vi "Periodic Tasks.vi"(8 "error in":errorcluster) -> ()   [LabVIEW 2020]
doc: "This VI runs in parallel to other tasks. It can contain as many user-defined periodic loops as you need. These can carry out PID or other sorts of timed response."
uses:
  myStates.ctl
  <vilib>/Rock Robotics/WPI/DriverStation/WPI_DriverStationRobotMode2.ctl
  4913f956-5bda-4107-8571-b517f3ac16c4.vi
  <vilib>/Rock Robotics/WPI/Utilities/WPI_GetSetVariantRefNum.vi
  <vilib>/Rock Robotics/Network Tables/NT Read Variant.vi
  <vilib>/Rock Robotics/Network Tables/NT Write Number.vi
  <vilib>/Rock Robotics/Network Tables/NT Read Number.vi
  Robot Global Data.vi
  <vilib>/Rock Robotics/Network Tables/NT Write Numeric Array.vi
  <vilib>/Rock Robotics/Network Tables/NT Write Boolean Array.vi
  <vilib>/Comparison/Equal/Equal Functor/Equal Functor.lvclass
  <vilib>/Rock Robotics/Network Tables/NT Write String.vi
  <vilib>/Utility/Data Type/NI_Data Type.lvlib
panel:
  in  "Current State":string
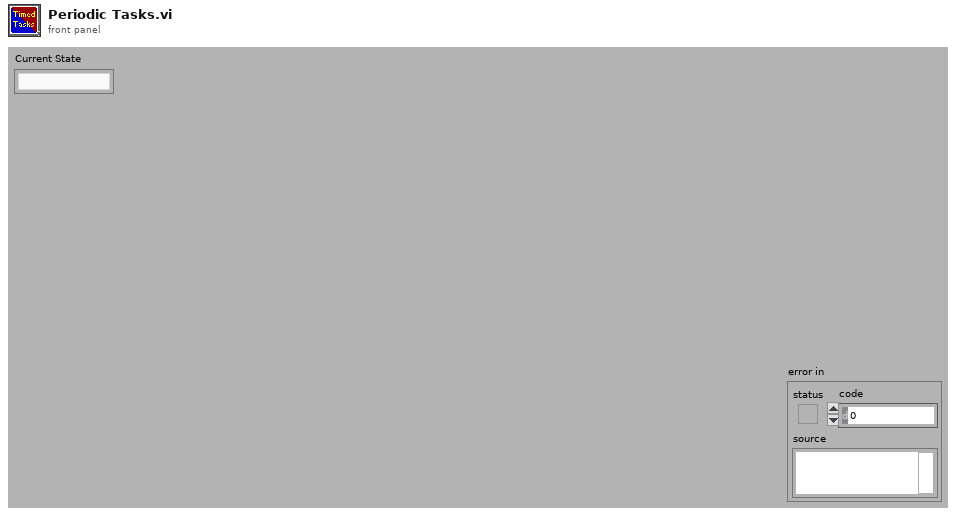
[diagram p1: front panel]
types:
  T1 = typedef "myStates.ctl" = enum16{"Init", "Manual Control", "Autonomous Traversal", "Avoid Left", "Avoid Right", "Return to Trench", "EXC Deploy", "EXC Excavate", "EXC Inch", "EXC Index", "EXC Retract", "Drive to Dep", "Approach Berm", "HAD Deploy", "HAD Deposit", "HAD Retract", "Return to EXC"}
  T2 = typedef "WPI_JoystickDevRef.ctl" = cluster{"Device":T3}
  T3 = typedef "WPI_JoystickDeviceEnum.ctl" = enum16{"USB 0", "USB 1", "USB 2", "USB 3", "USB 4", "USB 5"}
  T4 = typedef "WPI_RobotDriveDevRef.ctl" = cluster{"DevStatus":errorcluster, "Motors[]":T5[], "Square Inputs":bool, "Max Output":dbl}
  T5 = typedef "WPI_MotorControlDeviceRef.ctl" = cluster{"DeviceStatus":errorcluster, "Type":T6, "PWM":cluster{"PWM Channel":T7, "DeadBand":T8}, "CAN":cluster{"Device Number":u8, "SetOutput VI Ref":variant, "GetOutput VI Ref":variant, "Enable VI Ref":variant, "Disable VI Ref":variant, "Data":variant}, "Invert":bool, "DIO PWM":cluster{"PWM \"Enable\" Channel":T7, "DIOChannel":T9, "PWM Rate":dbl}}
  T6 = typedef "WPI_MotorControlType.ctl" = enum16{"PWM", "CAN", "DIO PWM"}
  T7 = typedef "FPGA_DIOPWMChannel.ctl" = enum8{"PWM 0", "PWM 1", "PWM 2", "PWM 3", "PWM 4", "PWM 5", "PWM 6", "PWM 7", "PWM 8", "PWM 9", "PWM MXP 0", "PWM MXP 1", "PWM MXP 2", "PWM MXP 3", "PWM MXP 4", "PWM MXP 5", "PWM MXP 6", "PWM MXP 7", "PWM MXP 8", "PWM MXP 9", "Invalid"}
  T8 = typedef "WPI_PWMDeadband.ctl" = cluster{"Name":string, "maxPositivePwm":i32, "minPositivePwm":i32, "centerPwm":i32, "maxNegativePwm":i32, "minNegativePwm":i32, "angularRange":u16}
  T9 = typedef "FPGA_DIOChannel.ctl" = enum8{"DIO 0", "DIO 1", "DIO 2", "DIO 3", "DIO 4", "DIO 5", "DIO 6", "DIO 7", "DIO 8", "DIO 9", "DIO MXP 0", "DIO MXP 1", "DIO MXP 2", "DIO MXP 3", "DIO MXP 4", "DIO MXP 5", "DIO MXP 6", "DIO MXP 7", "DIO MXP 8", "DIO MXP 9", "DIO MXP 10", "DIO MXP 11", "DIO MXP 12", "DIO MXP 13", "DIO MXP 14", "DIO MXP 15", "SPI Port CS1", "SPI Port CS2", "SPI Port CS3", "SPI Port MISO", "SPI Port MOSI", "Invalid"}
  T10 = cluster{"JoystickDevRef":T2, "RobotDriveDevRef":T4}
  T11 = typedef "WPI_DriverStationRobotMode2.ctl" = enum16{"Autonomous Disabled", "Autonomous Enabled", "Teleop Disabled", "Teleop Enabled", "Disconnected", "Finish", "Test Disabled", "Test Enabled", "Emergency Stopped"}
  T12 = cluster{"Axes[0]":dbl, "Axes[1]":dbl, "Axes[2]":dbl, "Axes[3]":dbl, "Axes[4]":dbl, "Axes[5]":dbl, "Axes[6]":dbl, "Axes[7]":dbl, "Axes[8]":dbl}
  T13 = cluster{"Buttons[0]":bool, "Buttons[1]":bool, "Buttons[2]":bool, "Buttons[3]":bool, "Buttons[4]":bool, "Buttons[5]":bool, "Buttons[6]":bool, "Buttons[7]":bool, "Buttons[8]":bool}
  T14 = typedef "WPI_AnalogChannelDevRef.ctl" = cluster{"DevStatus":errorcluster, "Analog Channel":T15}
  T15 = typedef "FPGA_AIChannel.ctl" = enum8{"AI 0", "AI 1", "AI 2", "AI 3", "AI MXP 0", "AI MXP 1", "AI MXP 2", "AI MXP 3", "Invalid"}
  T16 = typedef "WPI_DigitalOutputDevRef.ctl" = cluster{"DIO Channel":T9, "DevStatus":errorcluster}
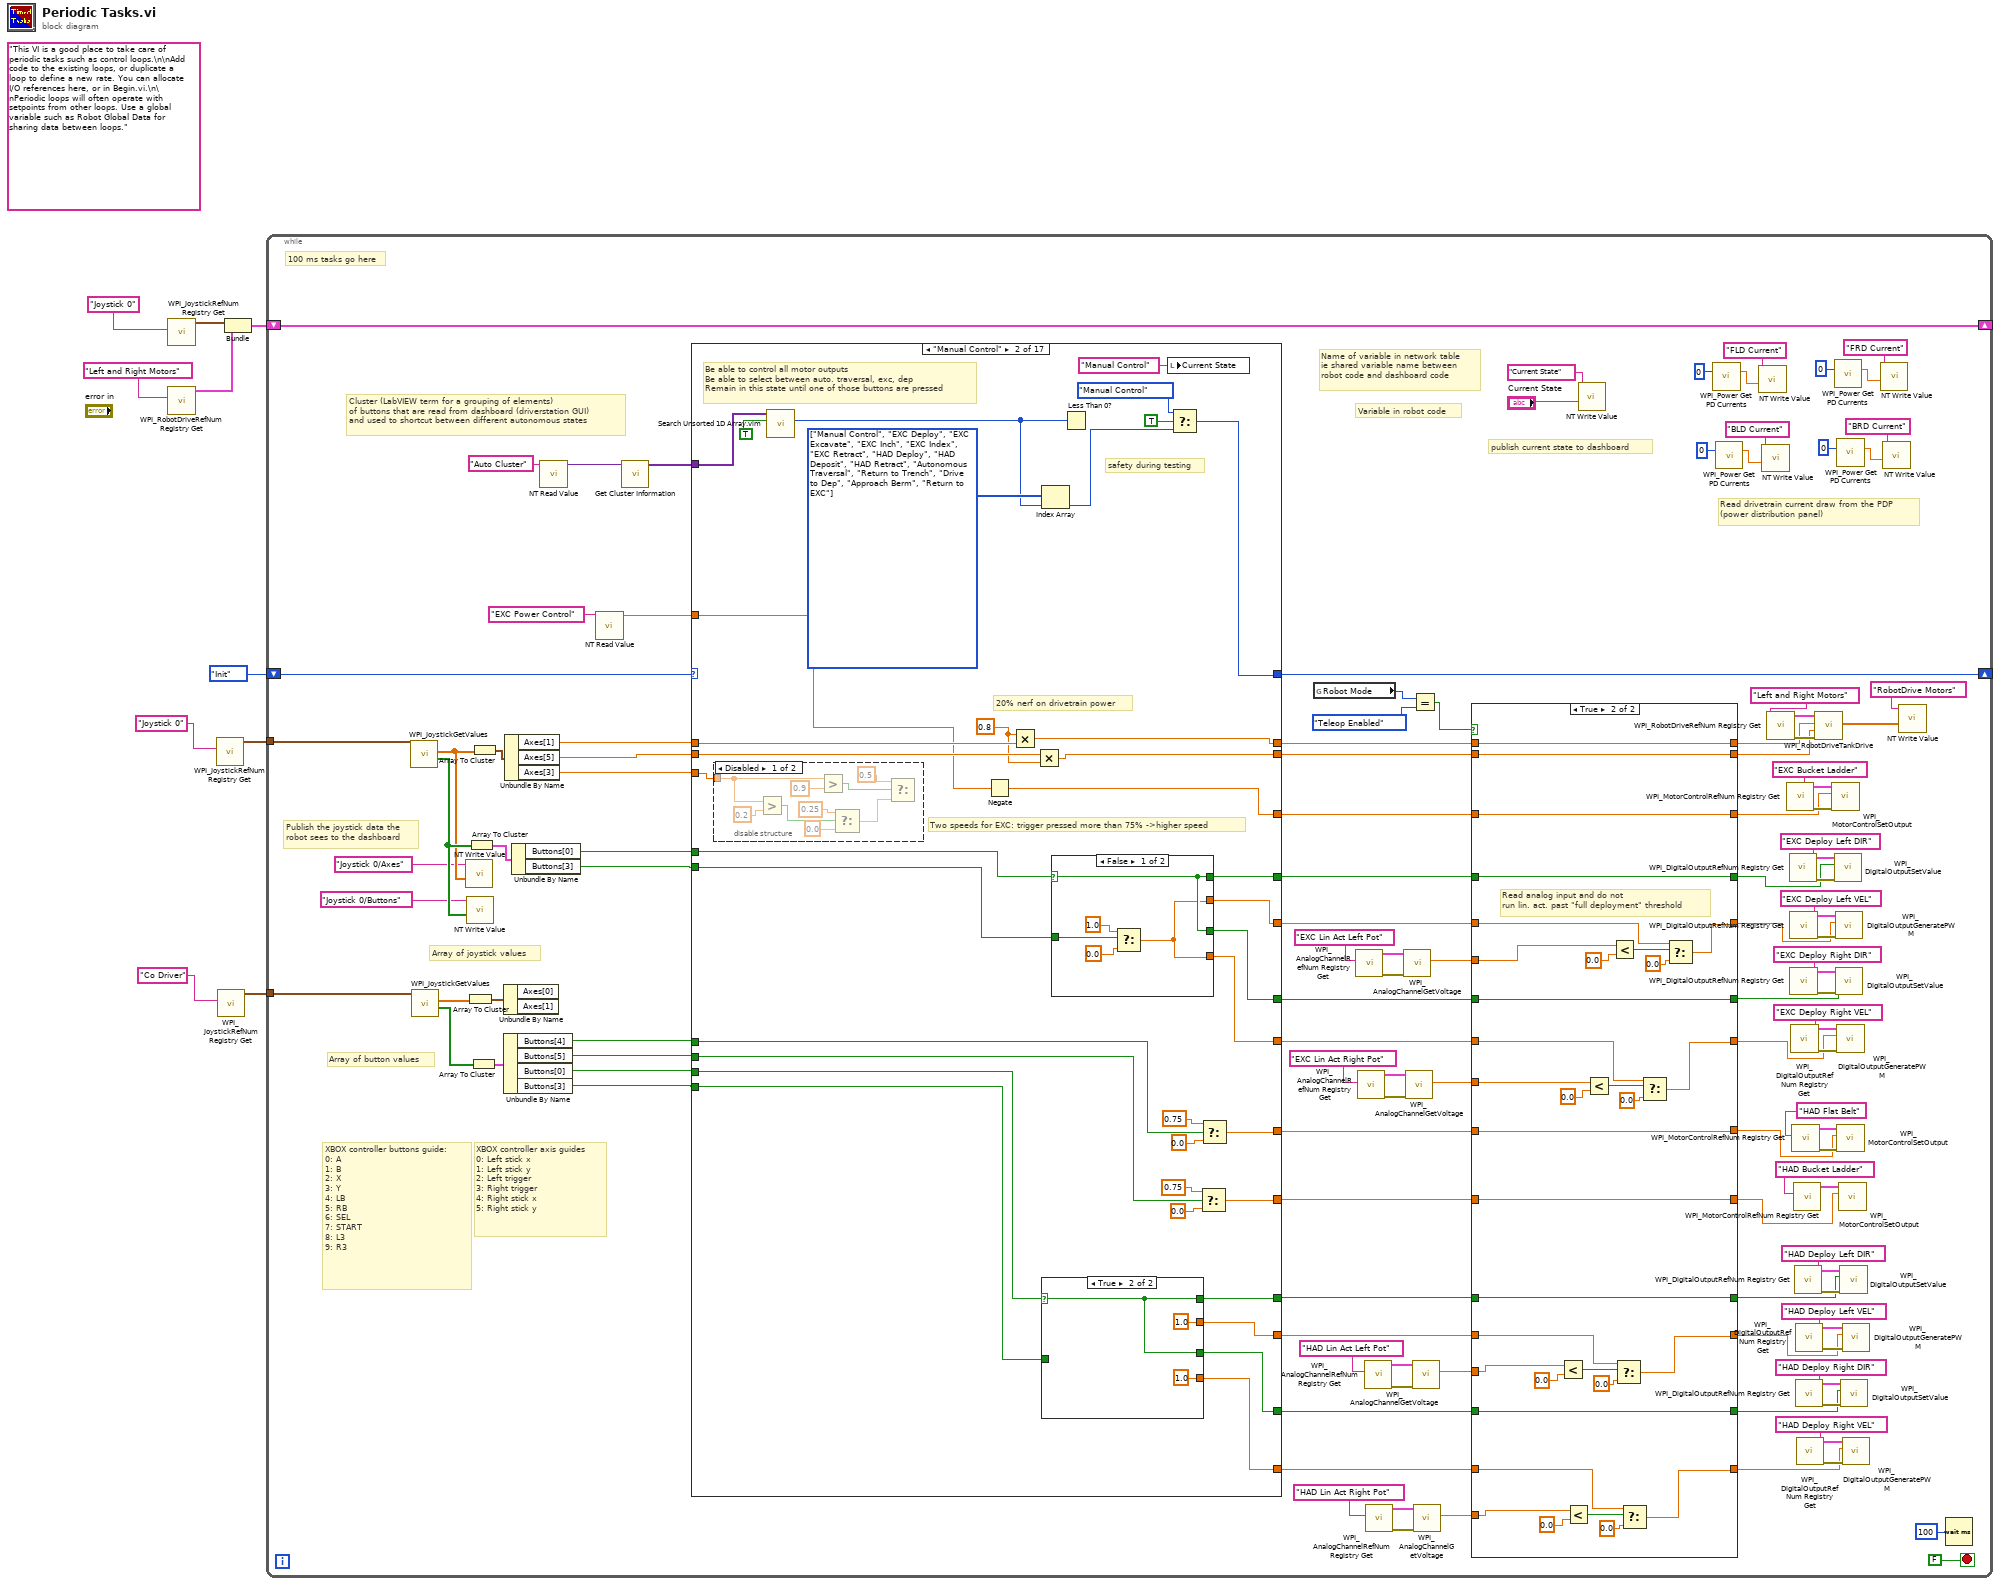
[diagram p0: block diagram]
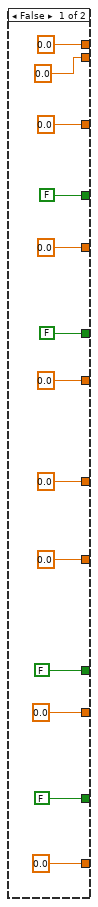
[diagram p2: hidden frame]
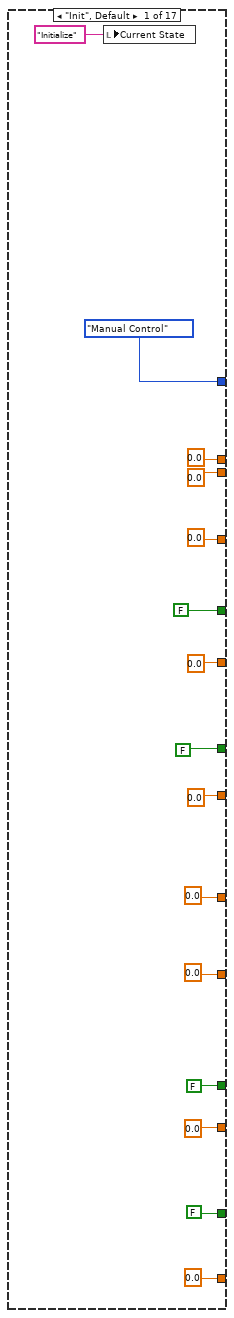
[diagram p3: hidden frame]
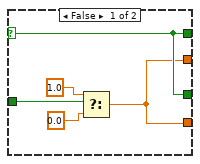
[diagram p5: hidden frame]
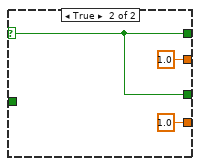
[diagram p6: hidden frame]
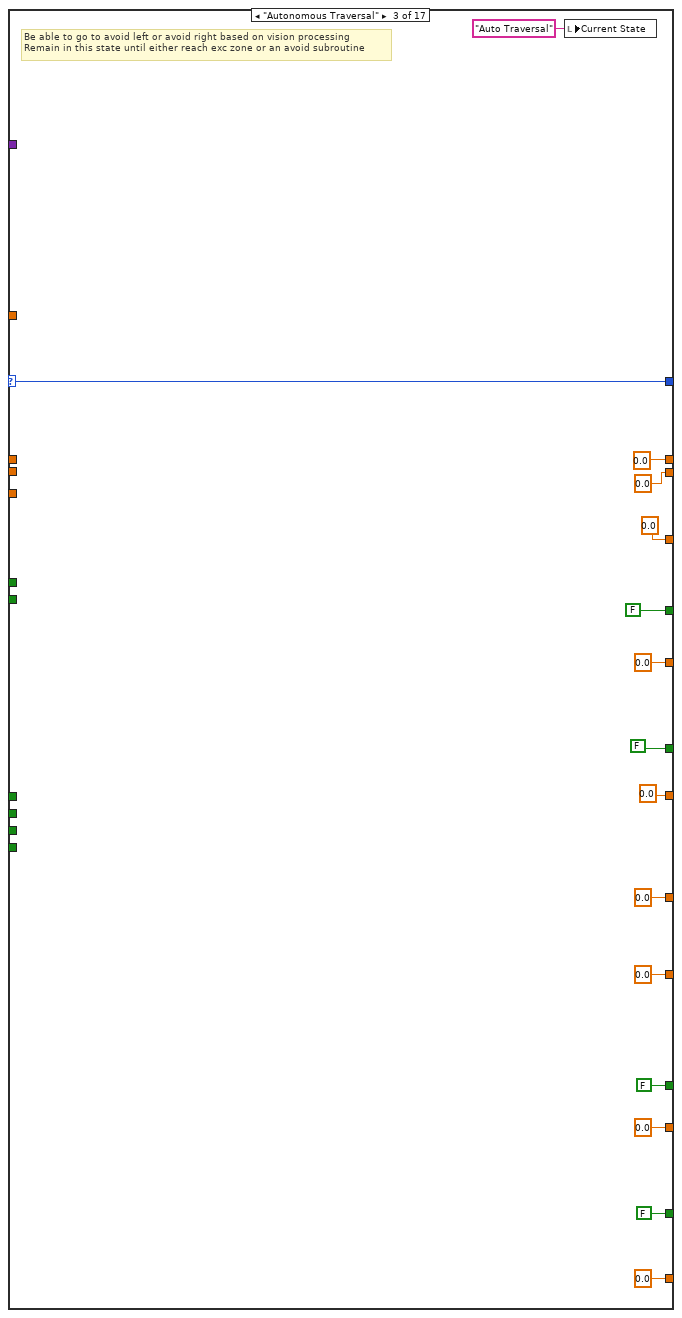
[diagram p7: hidden frame]
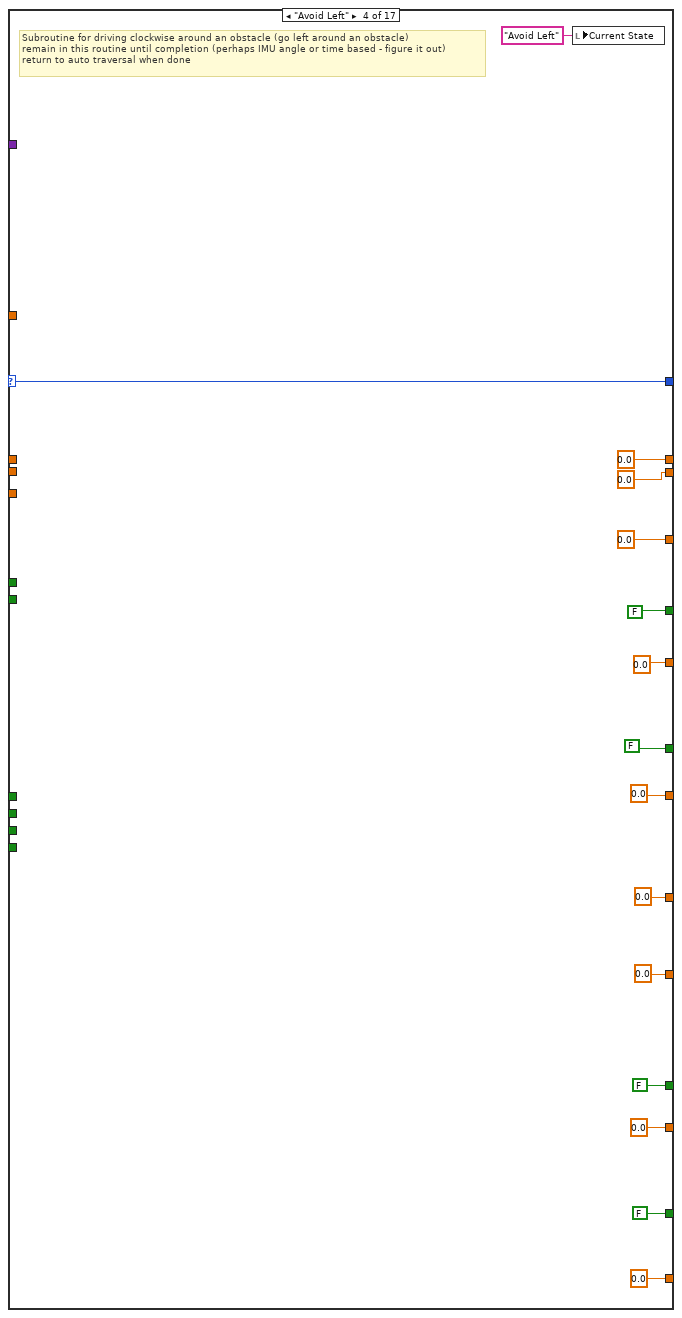
[diagram p8: hidden frame]
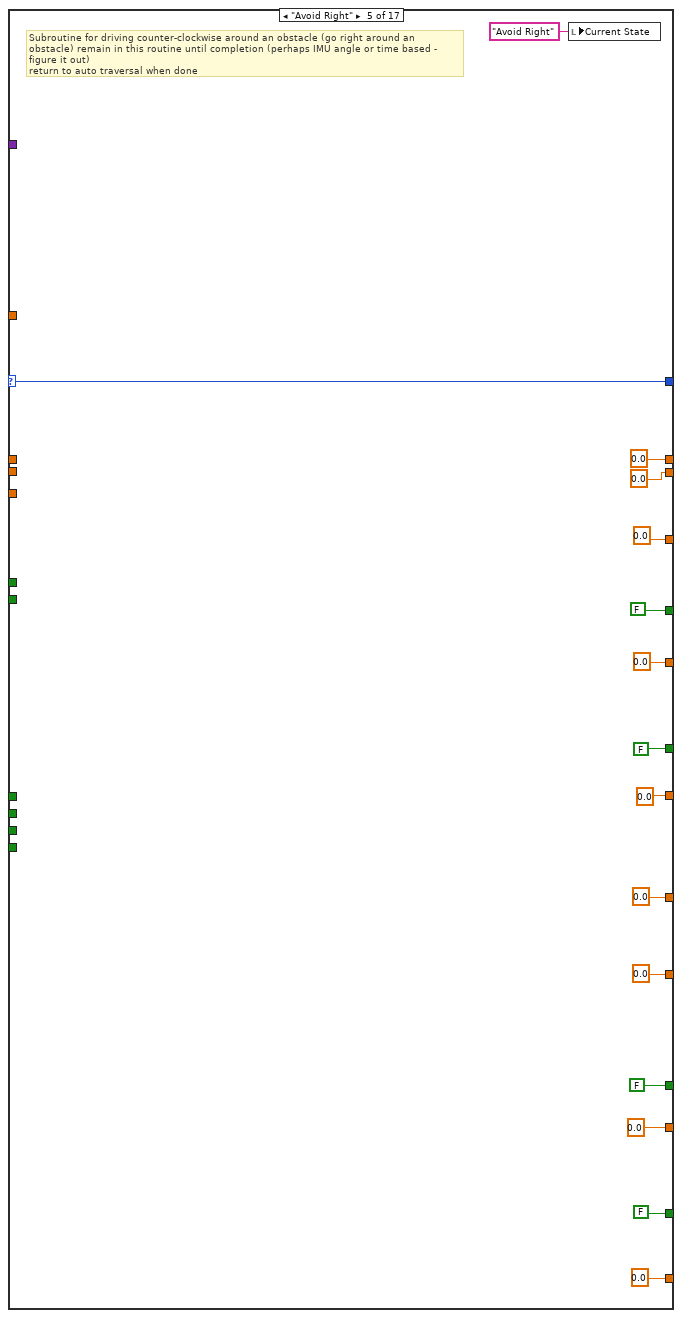
[diagram p9: hidden frame]
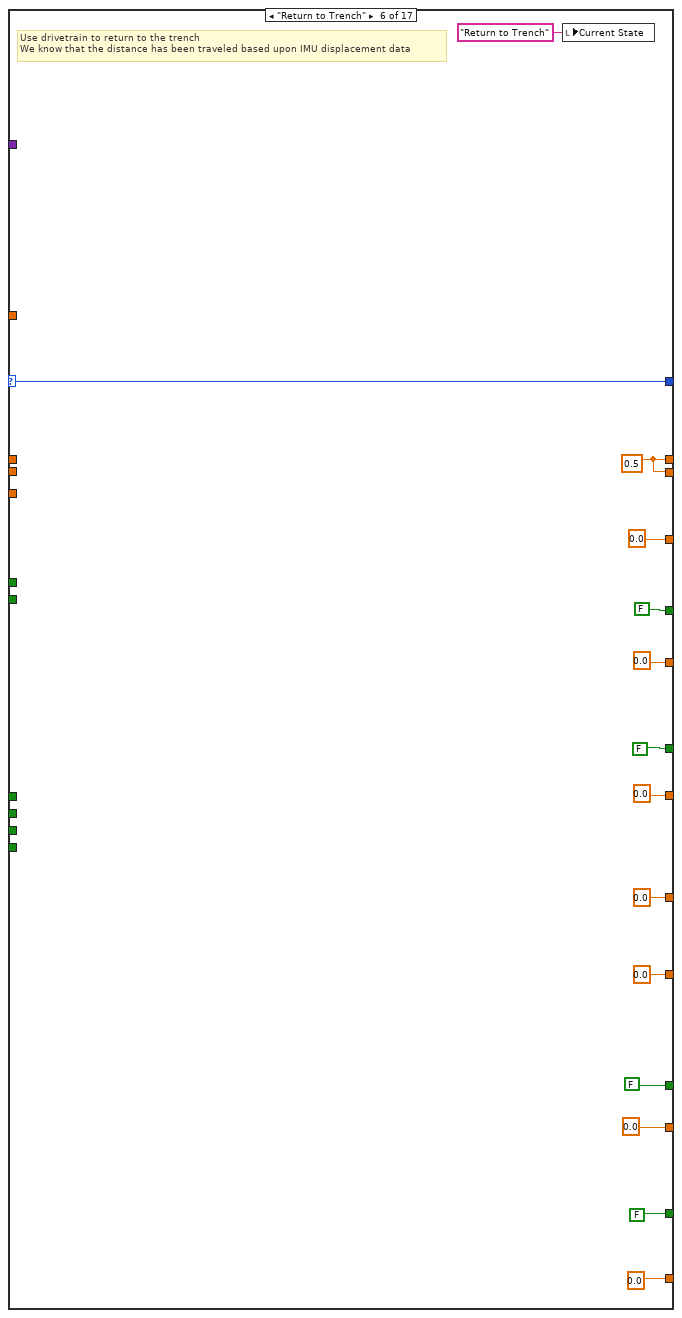
[diagram p10: hidden frame]
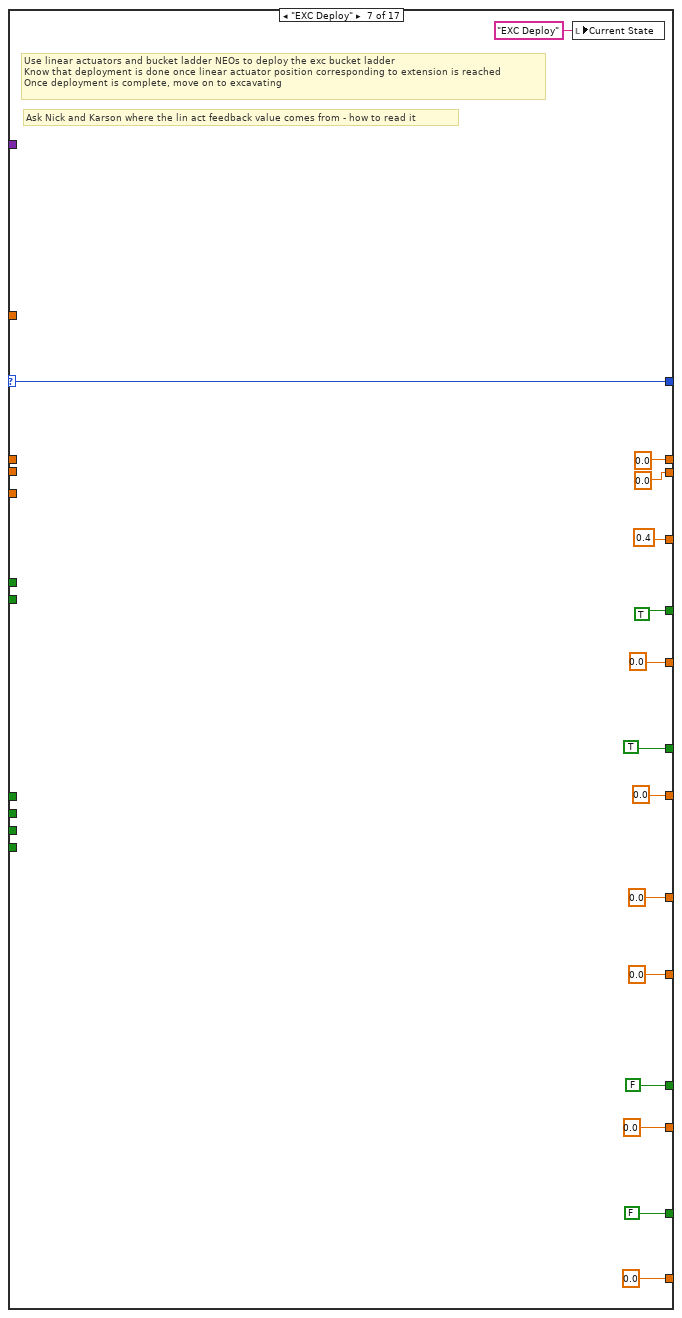
[diagram p11: hidden frame]
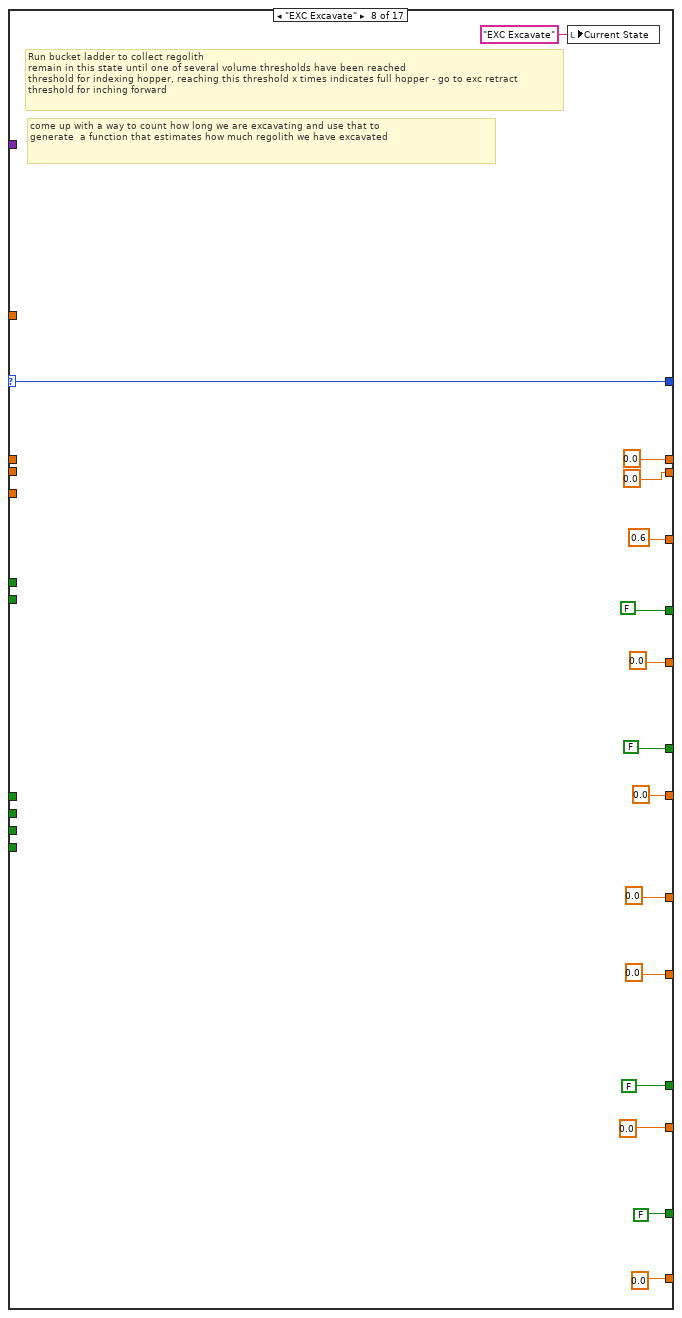
[diagram p12: hidden frame]
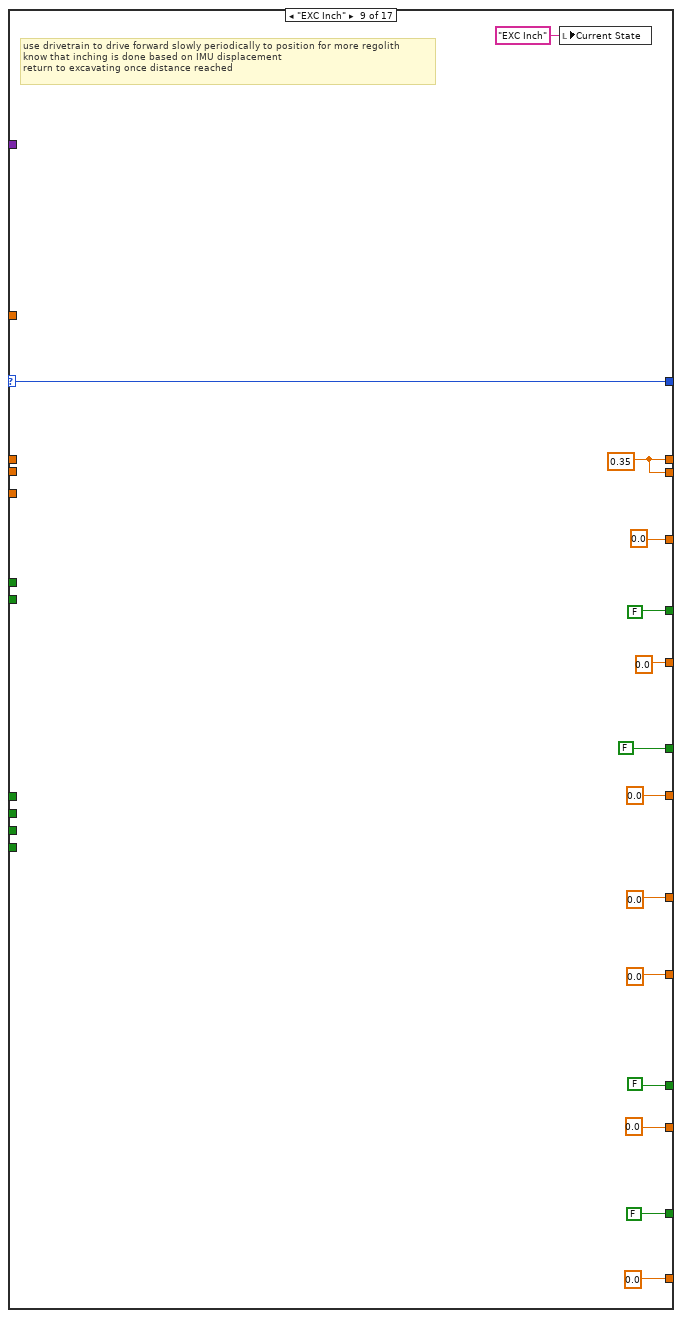
[diagram p13: hidden frame]
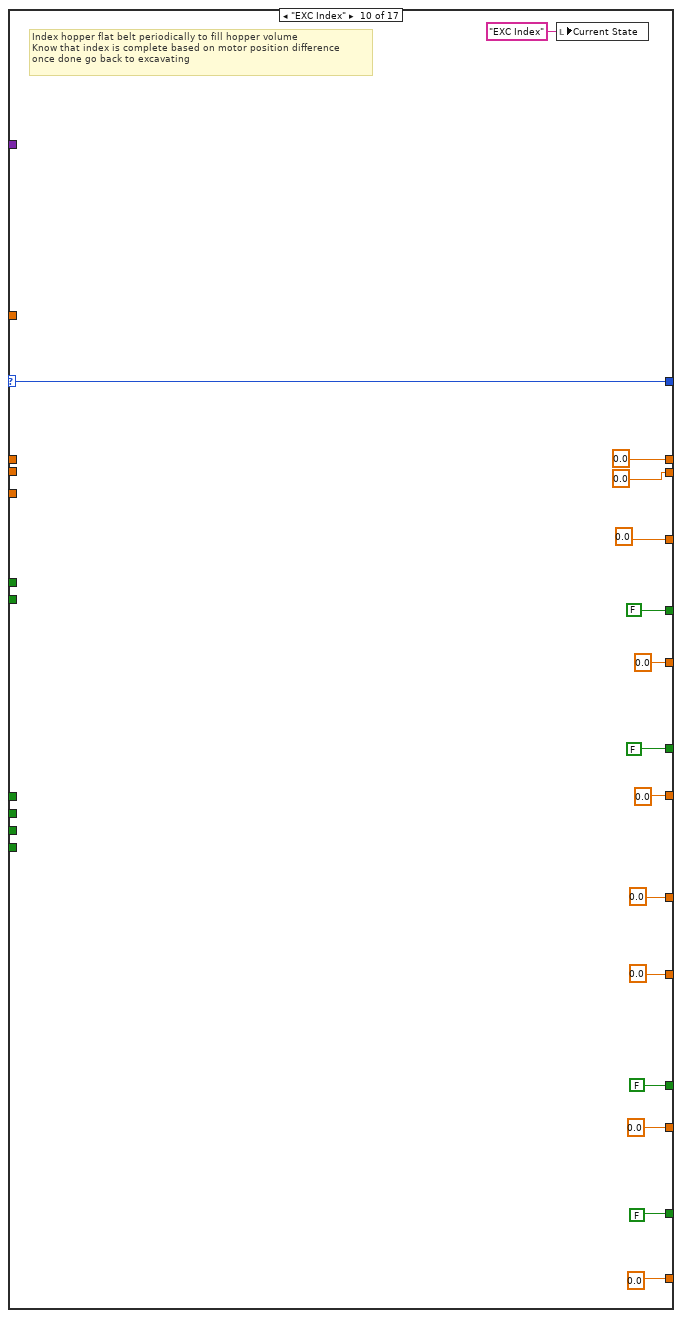
[diagram p14: hidden frame]
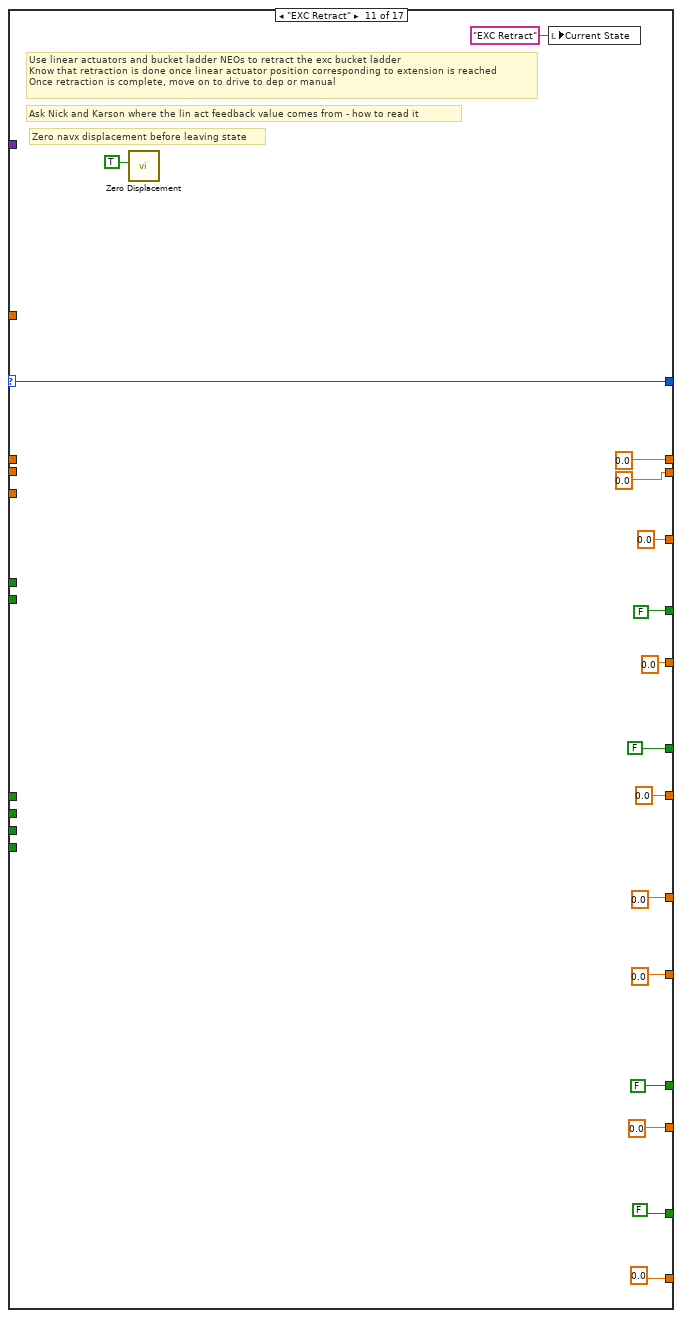
[diagram p15: hidden frame]
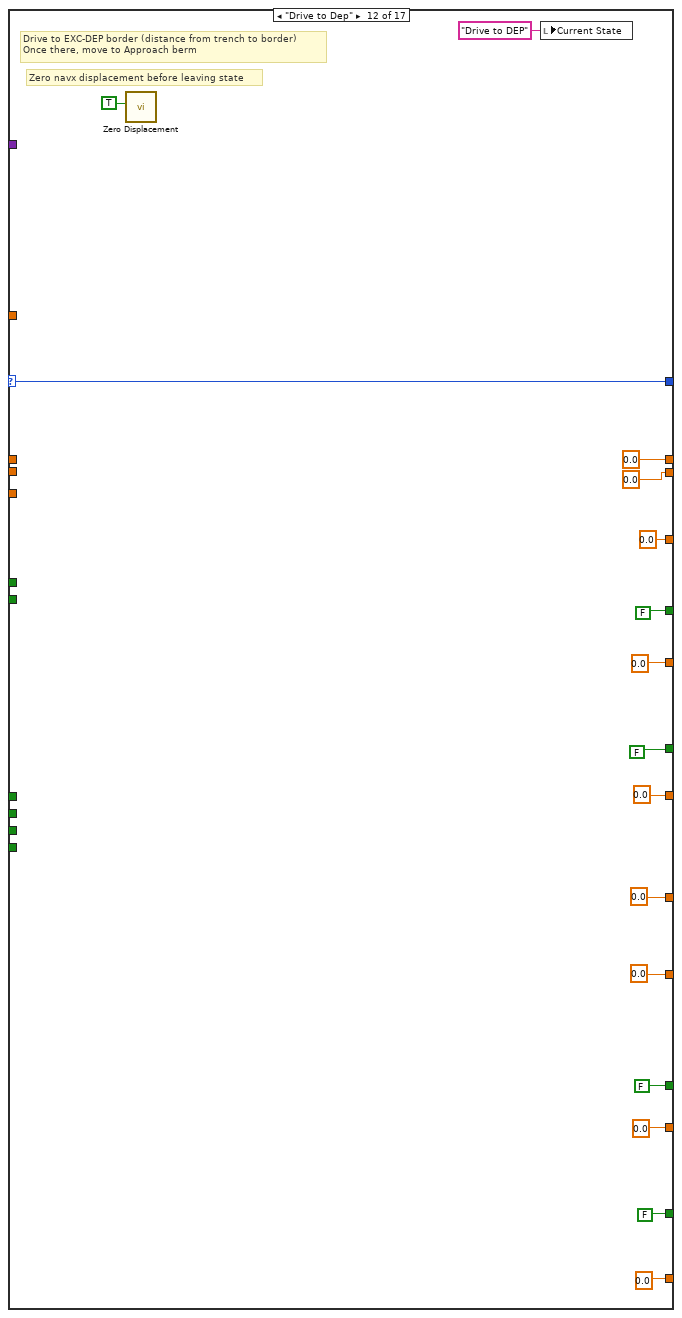
[diagram p16: hidden frame]
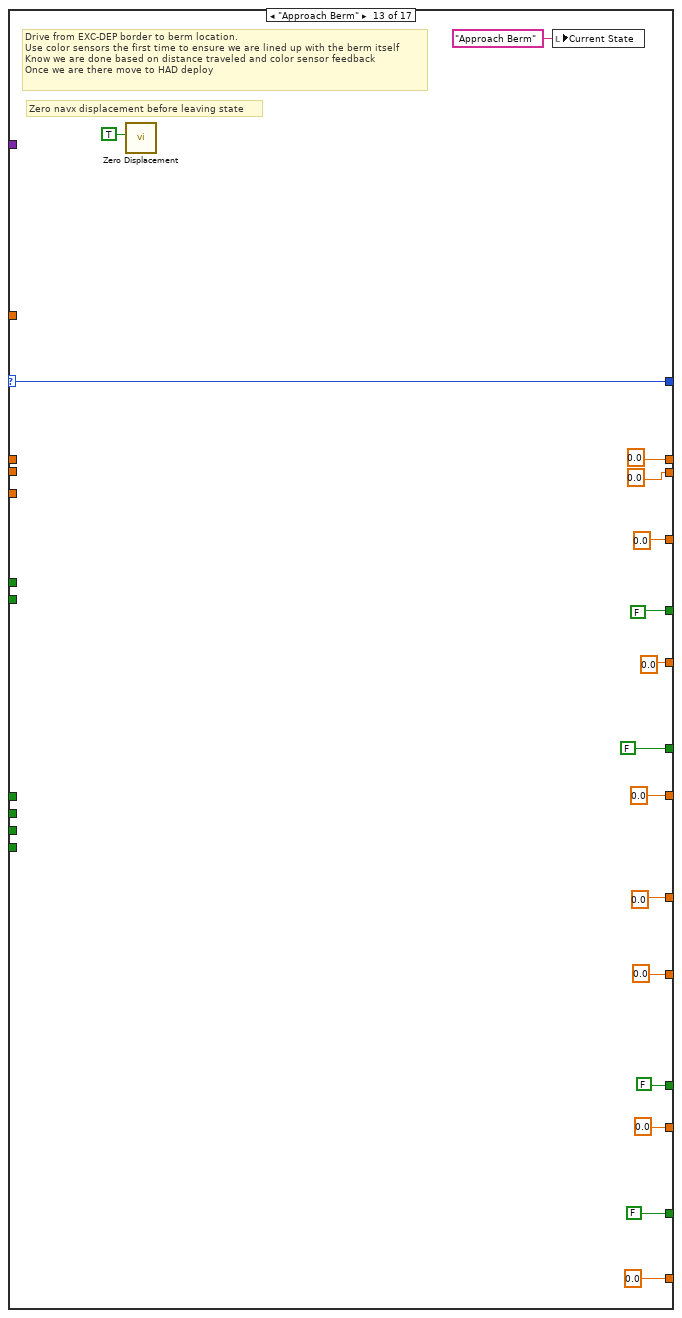
[diagram p17: hidden frame]
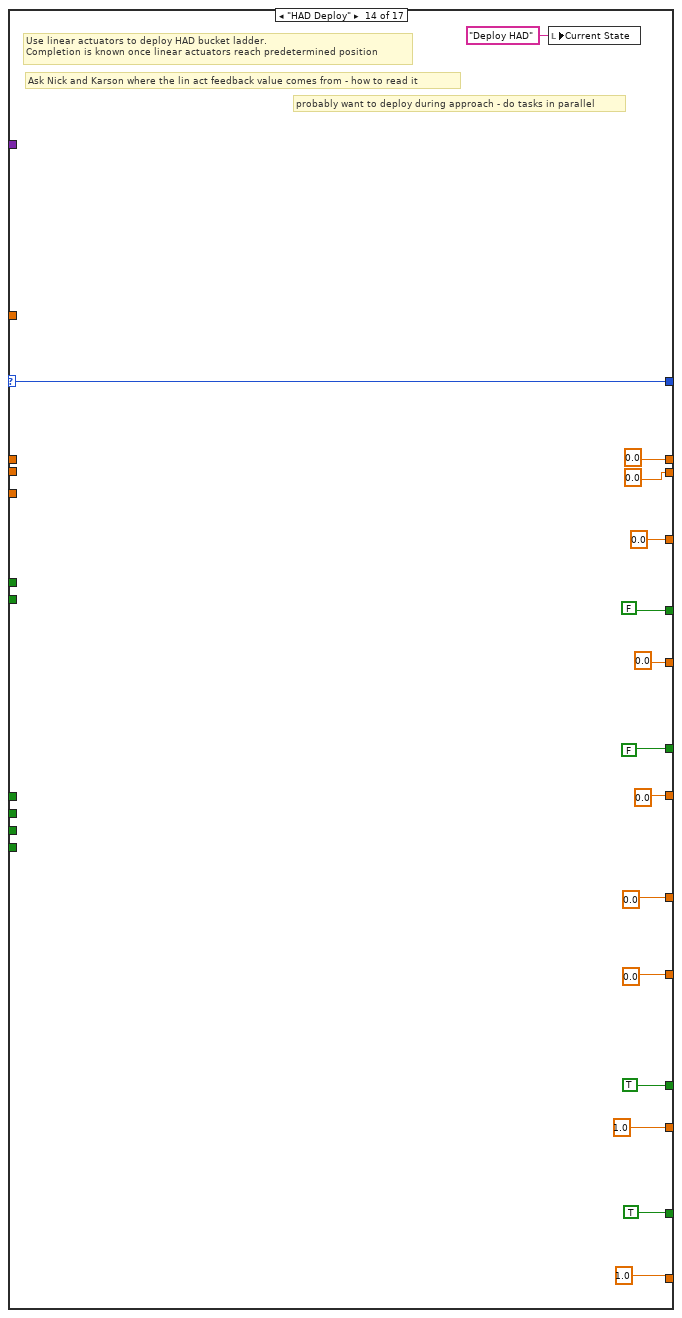
[diagram p18: hidden frame]
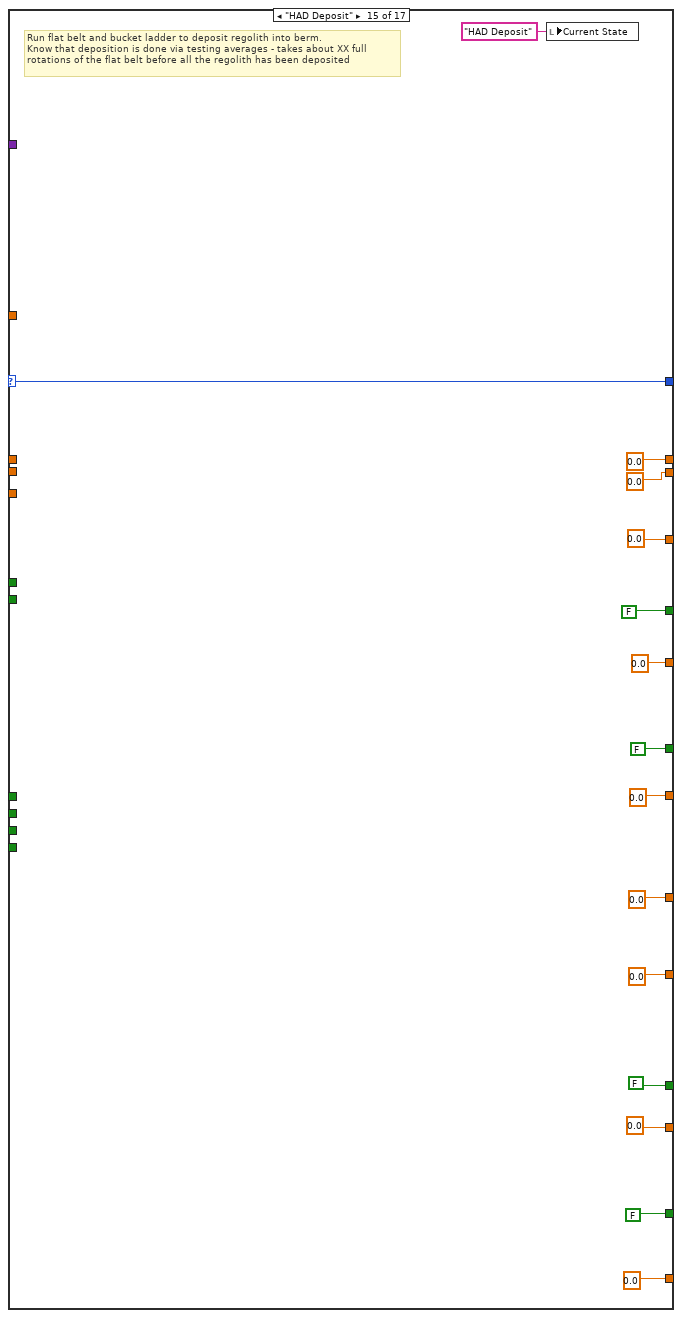
[diagram p19: hidden frame]
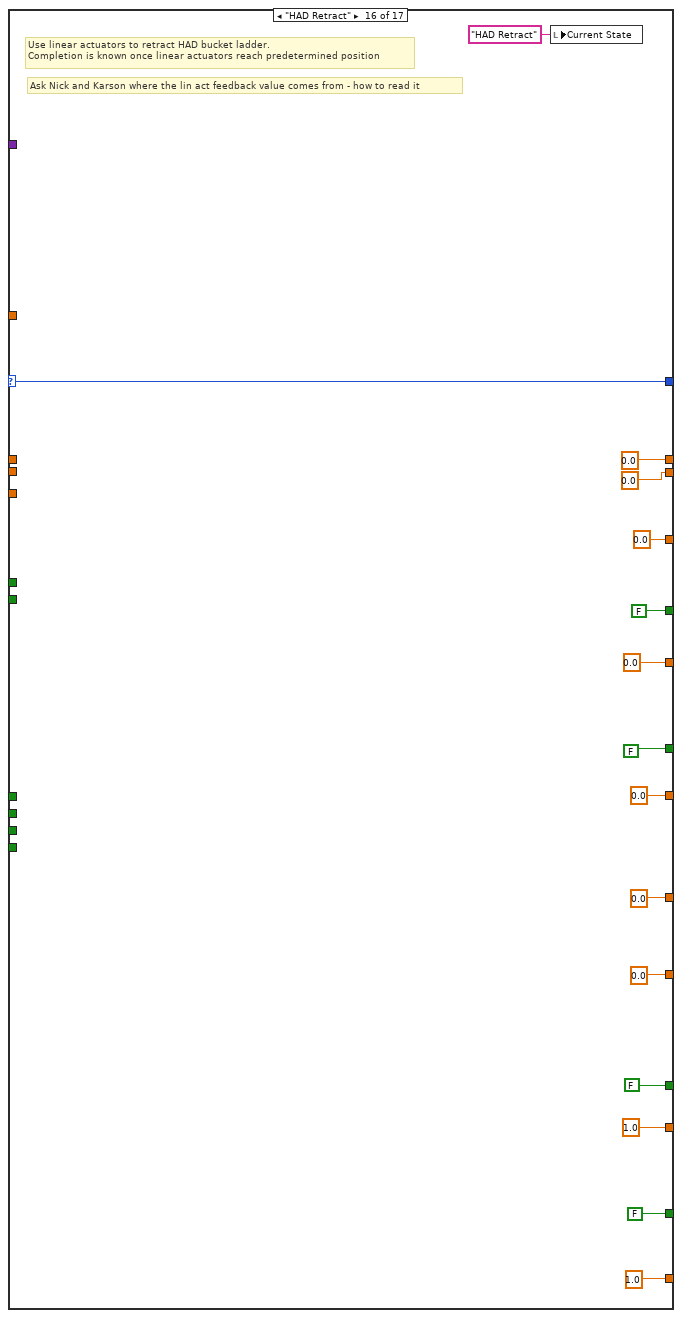
[diagram p20: hidden frame]
diagram:
  (unwired) "This VI is a good place to take care of periodic tasks such as control loops.\n\nAdd code to the existing loops, or duplicate a loop to define a new rate. You can allocate I/O references here, or in Begin.vi.\n\nPeriodic loops will often operate with setpoints from other loops. Use a global variable such as Robot Global Data for sharing data between loops."
  n1 = call <vilib>:"WPI_JoystickRefNum Registry Get.vi"("refnum name"="Joystick 0") -> ("JoystickDevRef"=w8:T2)  [unwired: 1 in, 9 out]
  n2 = call <vilib>:"WPI_RobotDriveRefNum Registry Get.vi"("refnum name"="Left and Right Motors") -> ("RobotDriveDevRef"=w7:T4)  [unwired: 1 in, 9 out]
  n3 = call <vilib>:"WPI_JoystickRefNum Registry Get.vi"("refnum name"="Joystick 0") -> ("JoystickDevRef"=w3:T2)  [unwired: 1 in, 9 out]
  n4 = call <vilib>:"WPI_JoystickRefNum Registry Get.vi"("refnum name"="Co Driver") -> ("JoystickDevRef"=w1:T2)  [unwired: 1 in, 9 out]
  n5 = Bundle("JoystickDevRef"=w8, "RobotDriveDevRef"=w7) -> (w6:T10)  [unwired: 1 out]
  n6 = while {
    shift-right: [w75] -> _
    shift-left: w6 -> [w75]
    shift-right: [w76] -> _
    shift-left: myStates."Init" -> [w77]
    tunnel: w3 -> [w74]
    tunnel: w1 -> [w73]
    stop <- FALSE stop-if-true
    # "Variable in robot code"
    # "Name of variable in network table\nie shared variable name between\nrobot code and dashboard code"
    # "publish current state to dashboard"
    # "Read drivetrain current draw from the PDP\n(power distribution panel)"
    # "XBOX controller axis guides\n0: Left stick x\n1: Left stick y\n2: Left trigger\n3: Right trigger\n4: Right stick x\n5: Right stick y"
    # "XBOX controller buttons guide:\n0: A\n1: B\n2: X\n3: Y\n4: LB\n5: RB\n6: SEL\n7: START\n8: L3\n9: R3"
    # "Array of joystick values"
    # "Array of button values"
    # "Cluster (LabVIEW term for a grouping of elements)\nof buttons that are read from dashboard (driverstation GUI)\nand used to shortcut between different autonomous states"
    # "Publish the joystick data the\nrobot sees to the dashboard"
    # "100 ms tasks go here"
    n7 = call <vilib>:"WPI_JoystickGetValues.vi"("JoystickDevRef"=w74) -> ("Buttons"=w94:bool[], "Axes"=w92:dbl[])  [unwired: 6 in, 3 out]
    n8 = call <vilib>:"WPI_JoystickGetValues.vi"("JoystickDevRef"=w73) -> ("Buttons"=w97:bool[], "Axes"=w99:dbl[])  [unwired: 6 in, 3 out]
    n9 = call-poly <vilib>:"NT Write Value.vi"("value"=w92, "name"="Joystick 0/Axes" ("Name")) -> ()  [unwired: 9 in, 1 out]
    n10 = call-poly <vilib>:"NT Write Value.vi"("value"=w94, "name"="Joystick 0/Buttons" ("Name")) -> ()  [unwired: 9 in, 1 out]
    n11 = Array To Cluster(array=w99) -> (cluster=w98:T12)
    n12 = Array To Cluster(array=w94) -> (cluster=w95:T13)
    n13 = Array To Cluster(array=w97) -> (cluster=w96:T13)
    n14 = Array To Cluster(array=w92) -> (cluster=w93:T12)
    n15 = Unbundle By Name(w98) -> ()  [unwired: 2 out]
    n16 = Unbundle By Name(w96) -> ("Buttons[4]"=w88:bool, "Buttons[5]"=w87:bool, "Buttons[0]"=w86:bool, "Buttons[3]"=w85:bool)
    n17 = Unbundle By Name(w93) -> ("Axes[1]"=w81:dbl, "Axes[5]"=w89:dbl, "Axes[3]"=w82:dbl)
    n18 = Unbundle By Name(w95) -> ("Buttons[0]"=w84:bool, "Buttons[3]"=w83:bool)
    n19 = call-poly <vilib>:"NT Read Value.vi"("name"="Auto Cluster") -> ("Variant"=w79:variant)  [unwired: 9 in, 1 out]
    n20 = call-poly <vilib>:"NT Read Value.vi"("name"="EXC Power Control") -> ("value"=w27:dbl)  [unwired: 8 in, 2 out]
    n21 = call <vilib>:"Get Cluster Information.vi"("variant"=w79) -> ("cluster elements"=w78:variant[])  [unwired: 9 in, 1 out]
    n22 = case shown="\"Manual Control\"" w77 {
      selector: w77 -> [_ _ w262 w277 w292 w307 w321 w336 w351 w365 w380 w396 w412 w428 w443 w458 w473]
      tunnel: [myStates."Manual Control" w203 w262 w277 w292 w307 w321 w336 w351 w365 w380 w396 w412 w428 w443 w458 w473] -> w76
      tunnel: [0.0 ("Output") w200 0.0 ("Output") 0.0 ("Output") 0.0 ("Output") 0.0 ("Output") 0.4 ("Output") 0.6 ("Output") 0.0 ("Output") 0.0 ("Output") 0.0 ("Output") 0.0 ("Output") 0.0 ("Output") 0.0 ("Output") 0.0 ("Output") 0.0 ("Output") 0.0 ("Output")] -> w69
      tunnel: [0.0 ("Left axis value") w235 0.0 ("Left axis value") 0.0 ("Left axis value") 0.0 ("Left axis value") w316 0.0 ("Left axis value") 0.0 ("Left axis value") w360 0.0 ("Left axis value") 0.0 ("Left axis value") 0.0 ("Left axis value") 0.0 ("Left axis value") 0.0 ("Left axis value") 0.0 ("Left axis value") 0.0 ("Left axis value") 0.0 ("Left axis value")] -> w71
      tunnel: [0.0 ("Right axis value") w231 0.0 ("Right axis value") 0.0 ("Right axis value") 0.0 ("Right axis value") w316 0.0 ("Right axis value") 0.0 ("Right axis value") w360 0.0 ("Right axis value") 0.0 ("Right axis value") 0.0 ("Right axis value") 0.0 ("Right axis value") 0.0 ("Right axis value") 0.0 ("Right axis value") 0.0 ("Right axis value") 0.0 ("Right axis value")] -> w70
      tunnel: w81 -> [_ w234 _ _ _ _ _ _ _ _ _ _ _ _ _ _ _]
      tunnel: w89 -> [_ w233 _ _ _ _ _ _ _ _ _ _ _ _ _ _ _]
      tunnel: w82 -> [_ w230 _ _ _ _ _ _ _ _ _ _ _ _ _ _ _]
      tunnel: w84 -> [_ w221 _ _ _ _ _ _ _ _ _ _ _ _ _ _ _]
      tunnel: w83 -> [_ w220 _ _ _ _ _ _ _ _ _ _ _ _ _ _ _]
      tunnel: w88 -> [_ w225 _ _ _ _ _ _ _ _ _ _ _ _ _ _ _]
      tunnel: [FALSE ("Buttons[0]") w219 FALSE ("Buttons[0]") FALSE ("Buttons[0]") FALSE ("Buttons[0]") FALSE ("Buttons[0]") TRUE ("Buttons[0]") FALSE ("Buttons[0]") FALSE ("Buttons[0]") FALSE ("Buttons[0]") FALSE ("Buttons[0]") FALSE ("Buttons[0]") FALSE ("Buttons[0]") FALSE ("Buttons[0]") FALSE ("Buttons[0]") FALSE ("Buttons[0]") FALSE ("Buttons[0]")] -> w68
      tunnel: w87 -> [_ w224 _ _ _ _ _ _ _ _ _ _ _ _ _ _ _]
      tunnel: [FALSE ("Buttons[1]") w216 FALSE ("Buttons[1]") FALSE ("Buttons[1]") FALSE ("Buttons[1]") FALSE ("Buttons[1]") TRUE ("Buttons[1]") FALSE ("Buttons[1]") FALSE ("Buttons[1]") FALSE ("Buttons[1]") FALSE ("Buttons[1]") FALSE ("Buttons[1]") FALSE ("Buttons[1]") FALSE ("Buttons[1]") FALSE ("Buttons[1]") FALSE ("Buttons[1]") FALSE ("Buttons[1]")] -> w66
      tunnel: [0.0 ("f") w217 0.0 ("f") 0.0 ("f") 0.0 ("f") 0.0 ("f") 0.0 ("f") 0.0 ("f") 0.0 ("f") 0.0 ("f") 0.0 ("f") 0.0 ("f") 0.0 ("f") 0.0 ("f") 0.0 ("f") 0.0 ("f") 0.0 ("f")] -> w65
      tunnel: [0.0 ("f") w218 0.0 ("f") 0.0 ("f") 0.0 ("f") 0.0 ("f") 0.0 ("f") 0.0 ("f") 0.0 ("f") 0.0 ("f") 0.0 ("f") 0.0 ("f") 0.0 ("f") 0.0 ("f") 0.0 ("f") 0.0 ("f") 0.0 ("f")] -> w67
      tunnel: [FALSE ("Value") w213 FALSE ("Value") FALSE ("Value") FALSE ("Value") FALSE ("Value") FALSE ("Value") FALSE ("Value") FALSE ("Value") FALSE ("Value") FALSE ("Value") FALSE ("Value") FALSE ("Value") TRUE ("Value") FALSE ("Value") FALSE ("Value") FALSE ("Value")] -> w62
      tunnel: [sgl 0.0 ("PWM Duty Cycle") w211 sgl 0.0 ("PWM Duty Cycle") sgl 0.0 ("PWM Duty Cycle") sgl 0.0 ("PWM Duty Cycle") sgl 0.0 ("PWM Duty Cycle") sgl 0.0 ("PWM Duty Cycle") sgl 0.0 ("PWM Duty Cycle") sgl 0.0 ("PWM Duty Cycle") sgl 0.0 ("PWM Duty Cycle") sgl 0.0 ("PWM Duty Cycle") sgl 0.0 ("PWM Duty Cycle") sgl 0.0 ("PWM Duty Cycle") sgl 1.0 ("PWM Duty Cycle") sgl 0.0 ("PWM Duty Cycle") sgl 1.0 ("PWM Duty Cycle") sgl 0.0 ("PWM Duty Cycle")] -> w61
      tunnel: [FALSE ("Value") w212 FALSE ("Value") FALSE ("Value") FALSE ("Value") FALSE ("Value") FALSE ("Value") FALSE ("Value") FALSE ("Value") FALSE ("Value") FALSE ("Value") FALSE ("Value") FALSE ("Value") TRUE ("Value") FALSE ("Value") FALSE ("Value") FALSE ("Value")] -> w60
      tunnel: [sgl 0.0 ("PWM Duty Cycle") w210 sgl 0.0 ("PWM Duty Cycle") sgl 0.0 ("PWM Duty Cycle") sgl 0.0 ("PWM Duty Cycle") sgl 0.0 ("PWM Duty Cycle") sgl 0.0 ("PWM Duty Cycle") sgl 0.0 ("PWM Duty Cycle") sgl 0.0 ("PWM Duty Cycle") sgl 0.0 ("PWM Duty Cycle") sgl 0.0 ("PWM Duty Cycle") sgl 0.0 ("PWM Duty Cycle") sgl 0.0 ("PWM Duty Cycle") sgl 1.0 ("PWM Duty Cycle") sgl 0.0 ("PWM Duty Cycle") sgl 1.0 ("PWM Duty Cycle") sgl 0.0 ("PWM Duty Cycle")] -> w59
      tunnel: [0.0 ("f") w223 0.0 ("f") 0.0 ("f") 0.0 ("f") 0.0 ("f") 0.0 ("f") 0.0 ("f") 0.0 ("f") 0.0 ("f") 0.0 ("f") 0.0 ("f") 0.0 ("f") 0.0 ("f") 0.0 ("f") 0.0 ("f") 0.0 ("f")] -> w64
      tunnel: [0.0 ("f") w222 0.0 ("f") 0.0 ("f") 0.0 ("f") 0.0 ("f") 0.0 ("f") 0.0 ("f") 0.0 ("f") 0.0 ("f") 0.0 ("f") 0.0 ("f") 0.0 ("f") 0.0 ("f") 0.0 ("f") 0.0 ("f") 0.0 ("f")] -> w63
      tunnel: w86 -> [_ w215 _ _ _ _ _ _ _ _ _ _ _ _ _ _ _]
      tunnel: w85 -> [_ w214 _ _ _ _ _ _ _ _ _ _ _ _ _ _ _]
      tunnel: w78 -> [_ w208 _ _ _ _ _ _ _ _ _ _ _ _ _ _ _]
      tunnel: w27 -> [_ w199 _ _ _ _ _ _ _ _ _ _ _ _ _ _ _]
      frame "Init", Default {
        n23 = local write "Current State"("Initialize" ("Current State")) -> ()
      }
      frame "Manual Control" {
        w206 = T1[] [enum."Manual Control", enum."EXC Deploy", enum."EXC Excavate", enum."EXC Inch", enum."EXC Index", enum."EXC Retract", enum."HAD Deploy", enum."HAD Deposit", enum."HAD Retract", enum."Autonomous Traversal", enum."Return to Trench", enum."Drive to Dep", enum."Approach Berm", enum."Return to EXC"] items=["Init", "Manual Control", "Autonomous Traversal", "Avoid Left", "Avoid Right", "Return to Trench", "EXC Deploy", "EXC Excavate", "EXC Inch", "EXC Index", "EXC Retract", "Drive to Dep", "Approach Berm", "HAD Deploy", "HAD Deposit", "HAD Retract", "Return to EXC"]
        w232 = 0.8 ("x")
        # "safety during testing"
        # "Two speeds for EXC: trigger pressed more than 75% ->higher speed"
        # "20% nerf on drivetrain power"
        # "Be able to control all motor outputs\nBe able to select between auto. traversal, exc, dep\nRemain in this state until one of those buttons are pressed"
        n24 = disable-structure shown="Disabled" {
          disable-tunnel: w230 -> [w241 _]
          frame Disabled {
            n25 = Greater?(x=w241, y=0.2) -> (0:w239:bool)
            n26 = Greater?(x=w241, y=0.9) -> (0:w243:bool)
            n27 = Select(t=0.25, s=w239, f=0.0) -> (s? t:f=w236:dbl)
            n28 = Select(t=0.5, s=w243, f=w236) -> ()  [unwired: 1 out]
          }
          frame Enabled {
          }
        }
        n29 = call "Search Unsorted 1D Array.vim"("element"=TRUE, "unsorted 1D array"=w208) -> ("index of element"=w205:i32)  [unwired: 9 in]
        n30 = Negate(x=w199) -> (-x=w200:dbl)
        n31 = Multiply(x=w232, y=w234) -> (x*y=w235:dbl)
        n32 = Multiply(x=w233, y=w232) -> (x*y=w231:dbl)
        n33 = Index Array(array=w206, index=w205) -> (element=w204:T1)
        n34 = case shown="True" w215 {
          selector: w215 -> [w249 w252]
          tunnel: w214 -> [w248 _]
          tunnel: [w249 w252] -> w213
          tunnel: [w245 1.0 ("f")] -> w211
          tunnel: [w245 1.0 ("f")] -> w210
          tunnel: [w249 w252] -> w212
          frame False {
            n35 = Select(t=1.0, s=w248, f=0.0) -> (s? t:f=w245:dbl)
          }
          frame True {
          }
        }
        n36 = case shown="False" w221 {
          selector: w221 -> [w257 w260]
          tunnel: w220 -> [w256 _]
          tunnel: [w257 w260] -> w219
          tunnel: [w253 1.0 ("f")] -> w218
          tunnel: [w253 1.0 ("f")] -> w217
          tunnel: [w257 w260] -> w216
          frame False {
            n37 = Select(t=1.0, s=w256, f=0.0) -> (s? t:f=w253:dbl)
          }
          frame True {
          }
        }
        n38 = Less Than 0?(x=w205) -> ()  [unwired: 1 out]
        n39 = local write "Current State"("Manual Control" ("Current State")) -> ()
        n40 = Select(t=myStates."Manual Control", s=TRUE, f=w204) -> (s? t:f=w203:T1)
        n41 = Select(t=0.75, s=w224, f=0.0) -> (s? t:f=w222:dbl)
        n42 = Select(t=0.75, s=w225, f=0.0) -> (s? t:f=w223:dbl)
      }
      frame "Autonomous Traversal" {
        # "Be able to go to avoid left or avoid right based on vision processing\nRemain in this state until either reach exc zone or an avoid subroutine"
        n43 = local write "Current State"("Auto Traversal" ("Current State")) -> ()
      }
      frame "Avoid Left" {
        # "Subroutine for driving clockwise around an obstacle (go left around an obstacle)\nremain in this routine until completion (perhaps IMU angle or time based - figure it out)\nreturn to auto traversal when done"
        n44 = local write "Current State"("Avoid Left" ("Current State")) -> ()
      }
      frame "Avoid Right" {
        # "Subroutine for driving counter-clockwise around an obstacle (go right around an obstacle) remain in this routine until completion (perhaps IMU angle or time based - figure it out)\nreturn to auto traversal when done"
        n45 = local write "Current State"("Avoid Right" ("Current State")) -> ()
      }
      frame "Return to Trench" {
        w316 = 0.5 ("Left axis value")
        # "Use drivetrain to return to the trench\nWe know that the distance has been traveled based upon IMU displacement data"
        n46 = local write "Current State"("Return to Trench" ("Current State")) -> ()
      }
      frame "EXC Deploy" {
        # "Ask Nick and Karson where the lin act feedback value comes from - how to read it"
        # "Use linear actuators and bucket ladder NEOs to deploy the exc bucket ladder\nKnow that deployment is done once linear actuator position corresponding to extension is reached\nOnce deployment is complete, move on to excavating"
        n47 = local write "Current State"("EXC Deploy" ("Current State")) -> ()
      }
      frame "EXC Excavate" {
        # "come up with a way to count how long we are excavating and use that to \ngenerate  a function that estimates how much regolith we have excavated"
        # "Run bucket ladder to collect regolith\nremain in this state until one of several volume thresholds have been reached\nthreshold for indexing hopper, reaching this threshold x times indicates full hopper - go to exc retract\nthreshold for inching forward"
        n48 = local write "Current State"("EXC Excavate" ("Current State")) -> ()
      }
      frame "EXC Inch" {
        w360 = 0.35 ("Left axis value")
        # "use drivetrain to drive forward slowly periodically to position for more regolith\nknow that inching is done based on IMU displacement\nreturn to excavating once distance reached"
        n49 = local write "Current State"("EXC Inch" ("Current State")) -> ()
      }
      frame "EXC Index" {
        # "Index hopper flat belt periodically to fill hopper volume\nKnow that index is complete based on motor position difference\nonce done go back to excavating"
        n50 = local write "Current State"("EXC Index" ("Current State")) -> ()
      }
      frame "EXC Retract" {
        # "Zero navx displacement before leaving state"
        # "Ask Nick and Karson where the lin act feedback value comes from - how to read it"
        # "Use linear actuators and bucket ladder NEOs to retract the exc bucket ladder\nKnow that retraction is done once linear actuator position corresponding to extension is reached\nOnce retraction is complete, move on to drive to dep or manual"
        n51 = call <vilib>:"Zero Displacement.vi"("Zero"=TRUE) -> ()  [unwired: 11 in]
        n52 = local write "Current State"("EXC Retract" ("Current State")) -> ()
      }
      frame "Drive to Dep" {
        # "Zero navx displacement before leaving state"
        # "Drive to EXC-DEP border (distance from trench to border)\nOnce there, move to Approach berm"
        n53 = call <vilib>:"Zero Displacement.vi"("Zero"=TRUE) -> ()  [unwired: 11 in]
        n54 = local write "Current State"("Drive to DEP" ("Current State")) -> ()
      }
      frame "Approach Berm" {
        # "Zero navx displacement before leaving state"
        # "Drive from EXC-DEP border to berm location.\nUse color sensors the first time to ensure we are lined up with the berm itself\nKnow we are done based on distance traveled and color sensor feedback\nOnce we are there move to HAD deploy"
        n55 = call <vilib>:"Zero Displacement.vi"("Zero"=TRUE) -> ()  [unwired: 11 in]
        n56 = local write "Current State"("Approach Berm" ("Current State")) -> ()
      }
      frame "HAD Deploy" {
        # "probably want to deploy during approach - do tasks in parallel"
        # "Ask Nick and Karson where the lin act feedback value comes from - how to read it"
        # "Use linear actuators to deploy HAD bucket ladder.\nCompletion is known once linear actuators reach predetermined position"
        n57 = local write "Current State"("Deploy HAD" ("Current State")) -> ()
      }
      frame "HAD Deposit" {
        # "Run flat belt and bucket ladder to deposit regolith into berm.\nKnow that deposition is done via testing averages - takes about XX full \nrotations of the flat belt before all the regolith has been deposited"
        n58 = local write "Current State"("HAD Deposit" ("Current State")) -> ()
      }
      frame "HAD Retract" {
        # "Ask Nick and Karson where the lin act feedback value comes from - how to read it"
        # "Use linear actuators to retract HAD bucket ladder.\nCompletion is known once linear actuators reach predetermined position"
        n59 = local write "Current State"("HAD Retract" ("Current State")) -> ()
      }
      frame "Return to EXC" {
        # "Drive back to EXC-DEP border using IMU distance data recorded during approach berm"
        n60 = local write "Current State"("Return to EXC" ("Current State")) -> ()
      }
    }
    n61 = global read "Robot Global Data.vi" "Robot Mode"() -> (w45:T11)
    n62 = call <vilib>:"WPI_AnalogChannelRefNum Registry Get.vi"("refnum name"="EXC Lin Act Left Pot") -> ("error out"=w25:errorcluster, "AIDeviceRef"=w26:T14)  [unwired: 9 in]
    n63 = call <vilib>:"WPI_AnalogChannelRefNum Registry Get.vi"("refnum name"="EXC Lin Act Right Pot") -> ("error out"=w21:errorcluster, "AIDeviceRef"=w20:T14)  [unwired: 9 in]
    n64 = call <vilib>:"WPI_AnalogChannelRefNum Registry Get.vi"("refnum name"="HAD Lin Act Left Pot") -> ("error out"=w17:errorcluster, "AIDeviceRef"=w18:T14)  [unwired: 9 in]
    n65 = call <vilib>:"WPI_AnalogChannelRefNum Registry Get.vi"("refnum name"="HAD Lin Act Right Pot") -> ("error out"=w13:errorcluster, "AIDeviceRef"=w12:T14)  [unwired: 9 in]
    n66 = call <vilib>:"WPI_AnalogChannelGetVoltage.vi"("error in (no error)"=w25, "AIDeviceRef"=w26) -> ("Voltage"=w23:dbl)  [unwired: 7 in, 2 out]
    n67 = call <vilib>:"WPI_AnalogChannelGetVoltage.vi"("error in (no error)"=w21, "AIDeviceRef"=w20) -> ("Voltage"=w19:dbl)  [unwired: 7 in, 2 out]
    n68 = Equal?(x=w45, y=WPI_DriverStationRobotMode2."Teleop Enabled") -> (x = y?=w43:bool)
    n69 = call <vilib>:"WPI_AnalogChannelGetVoltage.vi"("error in (no error)"=w17, "AIDeviceRef"=w18) -> ("Voltage"=w15:dbl)  [unwired: 7 in, 2 out]
    n70 = call <vilib>:"WPI_AnalogChannelGetVoltage.vi"("error in (no error)"=w13, "AIDeviceRef"=w12) -> ("Voltage"=w11:dbl)  [unwired: 7 in, 2 out]
    n71 = case shown="True" w43 {
      tunnel: [0.0 ("Left axis value") w183] -> w58
      tunnel: w71 -> [_ w183]
      tunnel: [0.0 ("Right axis value") w182] -> w57
      tunnel: w70 -> [_ w182]
      tunnel: [0.0 ("Output") w181] -> w56
      tunnel: w69 -> [_ w181]
      tunnel: [FALSE ("Buttons[0]") w180] -> w55
      tunnel: w68 -> [_ w180]
      tunnel: [0.0 ("f") w170] -> w54
      tunnel: w67 -> [_ w171]
      tunnel: [FALSE ("Buttons[1]") w179] -> w53
      tunnel: w66 -> [_ w179]
      tunnel: [0.0 ("f") w163] -> w52
      tunnel: w65 -> [_ w164]
      tunnel: [0.0 ("f") w178] -> w51
      tunnel: w64 -> [_ w178]
      tunnel: [0.0 ("f") w177] -> w50
      tunnel: w63 -> [_ w177]
      tunnel: [FALSE ("Value") w176] -> w49
      tunnel: w62 -> [_ w176]
      tunnel: [0.0 ("f") w151] -> w48
      tunnel: w61 -> [_ w152]
      tunnel: [FALSE ("Value") w175] -> w47
      tunnel: w60 -> [_ w175]
      tunnel: [0.0 ("f") w157] -> w46
      tunnel: w59 -> [_ w158]
      tunnel: w23 -> [_ w174]
      tunnel: w19 -> [_ w165]
      tunnel: w15 -> [_ w153]
      tunnel: w11 -> [_ w159]
      frame False {
      }
      frame True {
        # "Read analog input and do not\nrun lin. act. past \"full deployment\" threshold"
        n72 = Less?(x=w153, y=0.0) -> (x < y?=w155:bool)
        n73 = Less?(x=w159, y=0.0) -> (x < y?=w161:bool)
        n74 = Less?(x=w165, y=0.0) -> (x < y?=w167:bool)
        n75 = Less?(x=w174, y=0.0) -> (x < y?=w172:bool)
        n76 = Select(t=w152, s=w155, f=0.0) -> (s? t:f=w151:dbl)
        n77 = Select(t=w158, s=w161, f=0.0) -> (s? t:f=w157:dbl)
        n78 = Select(t=w164, s=w167, f=0.0) -> (s? t:f=w163:dbl)
        n79 = Select(t=w171, s=w172, f=0.0) -> (s? t:f=w170:dbl)
      }
    }
    n80 = call-poly <vilib>:"NT Write Value.vi"("value"="Current State", "name"="Current State") -> ()  [unwired: 9 in, 1 out]
    n81 = call <vilib>:"WPI_Power Get PD Currents.vi"("PD Channel"=0) -> ("current (A)"=w38:dbl)  [unwired: 11 in, 3 out]
    n82 = call <vilib>:"WPI_Power Get PD Currents.vi"("PD Channel"=0) -> ("current (A)"=w31:dbl)  [unwired: 11 in, 3 out]
    n83 = call-poly <vilib>:"NT Write Value.vi"("value"=w38, "name"="FLD Current") -> ()  [unwired: 9 in, 1 out]
    n84 = call-poly <vilib>:"NT Write Value.vi"("value"=w31, "name"="BLD Current") -> ()  [unwired: 9 in, 1 out]
    n85 = call <vilib>:"WPI_RobotDriveRefNum Registry Get.vi"("refnum name"="Left and Right Motors") -> ("error out"=w132:errorcluster, "RobotDriveDevRef"=w131:T4)  [unwired: 9 in]
    n86 = call <vilib>:"WPI_MotorControlRefNum Registry Get.vi"("refnum name"="EXC Bucket Ladder") -> ("error out"=w135:errorcluster, "MotorControlDevRef"=w134:T5)  [unwired: 9 in]
    n87 = call <vilib>:"WPI_DigitalOutputRefNum Registry Get.vi"("refnum name"="EXC Deploy Left DIR") -> ("error out"=w129:errorcluster, "DigitalOutputDevRef"=w128:T16)  [unwired: 9 in]
    n88 = call <vilib>:"WPI_DigitalOutputRefNum Registry Get.vi"("refnum name"="EXC Deploy Left VEL") -> ("error out"=w101:errorcluster, "DigitalOutputDevRef"=w100:T16)  [unwired: 9 in]
    n89 = call <vilib>:"WPI_DigitalOutputRefNum Registry Get.vi"("refnum name"="EXC Deploy Right DIR") -> ("error out"=w122:errorcluster, "DigitalOutputDevRef"=w123:T16)  [unwired: 9 in]
    n90 = call <vilib>:"WPI_DigitalOutputRefNum Registry Get.vi"("refnum name"="EXC Deploy Right VEL") -> ("error out"=w119:errorcluster, "DigitalOutputDevRef"=w118:T16)  [unwired: 9 in]
    n91 = call <vilib>:"WPI_MotorControlRefNum Registry Get.vi"("refnum name"="HAD Flat Belt") -> ("error out"=w104:errorcluster, "MotorControlDevRef"=w105:T5)  [unwired: 9 in]
    n92 = call <vilib>:"WPI_MotorControlRefNum Registry Get.vi"("refnum name"="HAD Bucket Ladder") -> ("MotorControlDevRef"=w103:T5)  [unwired: 9 in, 1 out]
    n93 = call <vilib>:"WPI_DigitalOutputRefNum Registry Get.vi"("refnum name"="HAD Deploy Left DIR") -> ("error out"=w106:errorcluster, "DigitalOutputDevRef"=w107:T16)  [unwired: 9 in]
    n94 = call <vilib>:"WPI_DigitalOutputRefNum Registry Get.vi"("refnum name"="HAD Deploy Left VEL") -> ("error out"=w114:errorcluster, "DigitalOutputDevRef"=w115:T16)  [unwired: 9 in]
    n95 = call <vilib>:"WPI_DigitalOutputRefNum Registry Get.vi"("refnum name"="HAD Deploy Right DIR") -> ("error out"=w113:errorcluster, "DigitalOutputDevRef"=w112:T16)  [unwired: 9 in]
    n96 = call <vilib>:"WPI_DigitalOutputRefNum Registry Get.vi"("refnum name"="HAD Deploy Right VEL") -> ("error out"=w116:errorcluster, "DigitalOutputDevRef"=w117:T16)  [unwired: 9 in]
    n97 = call <vilib>:"WPI_RobotDriveTankDrive.vi"("error in (no error)"=w132, "Right axis value"=w57, "Left axis value"=w58, "RobotDriveDevRef"=w131) -> ("Motor Values"=w120:dbl[])  [unwired: 5 in, 2 out]
    n98 = call <vilib>:"WPI_MotorControlSetOutput.vi"("error in (no error)"=w135, "Output"=w56, "MotorControlDevRef"=w134) -> ()  [unwired: 6 in, 3 out]
    n99 = call <vilib>:"WPI_Power Get PD Currents.vi"("PD Channel"=0) -> ("current (A)"=w37:dbl)  [unwired: 11 in, 3 out]
    n100 = call <vilib>:"WPI_DigitalOutputSetValue.vi"("error in (no error)"=w129, "Value"=w55, "DigitalOutputDevRef"=w128) -> ()  [unwired: 7 in, 2 out]
    n101 = call <vilib>:"WPI_DigitalOutputGeneratePWM.vi"("error in (no error)"=w101, "PWM Duty Cycle"=w54, "DigitalOutputDevRef"=w100) -> ()  [unwired: 7 in, 2 out]
    n102 = call <vilib>:"WPI_DigitalOutputSetValue.vi"("error in (no error)"=w122, "Value"=w53, "DigitalOutputDevRef"=w123) -> ()  [unwired: 7 in, 2 out]
    n103 = call <vilib>:"WPI_Power Get PD Currents.vi"("PD Channel"=0) -> ("current (A)"=w32:dbl)  [unwired: 11 in, 3 out]
    n104 = call <vilib>:"WPI_DigitalOutputGeneratePWM.vi"("error in (no error)"=w119, "PWM Duty Cycle"=w52, "DigitalOutputDevRef"=w118) -> ()  [unwired: 7 in, 2 out]
    n105 = call <vilib>:"WPI_MotorControlSetOutput.vi"("error in (no error)"=w104, "Output"=w51, "MotorControlDevRef"=w105) -> ()  [unwired: 6 in, 3 out]
    n106 = call <vilib>:"WPI_MotorControlSetOutput.vi"("Output"=w50, "MotorControlDevRef"=w103) -> ()  [unwired: 7 in, 3 out]
    n107 = call <vilib>:"WPI_DigitalOutputSetValue.vi"("error in (no error)"=w106, "Value"=w49, "DigitalOutputDevRef"=w107) -> ()  [unwired: 7 in, 2 out]
    n108 = call <vilib>:"WPI_DigitalOutputSetValue.vi"("error in (no error)"=w113, "Value"=w47, "DigitalOutputDevRef"=w112) -> ()  [unwired: 7 in, 2 out]
    n109 = call <vilib>:"WPI_DigitalOutputGeneratePWM.vi"("error in (no error)"=w114, "PWM Duty Cycle"=w48, "DigitalOutputDevRef"=w115) -> ()  [unwired: 7 in, 2 out]
    n110 = call <vilib>:"WPI_DigitalOutputGeneratePWM.vi"("error in (no error)"=w116, "PWM Duty Cycle"=w46, "DigitalOutputDevRef"=w117) -> ()  [unwired: 7 in, 2 out]
    n111 = call-poly <vilib>:"NT Write Value.vi"("value"=w37, "name"="FRD Current") -> ()  [unwired: 9 in, 1 out]
    n112 = call-poly <vilib>:"NT Write Value.vi"("value"=w32, "name"="BRD Current") -> ()  [unwired: 9 in, 1 out]
    n113 = call-poly <vilib>:"NT Write Value.vi"("value"=w120, "name"="RobotDrive Motors" ("Name")) -> ()  [unwired: 9 in, 1 out]
    n114 = Wait (ms)(milliseconds to wait=u32 100) -> ()  [unwired: 1 out]
  }
